vi "Prepare Control.vi"(7 "VolatusAPI":refnum<class "VolatusAPI.lvclass">, 8 "error in (no error)":errorcluster, 11 "ValveControl in":refnum<class "DigitalControl.lvclass">) -> (0 "error out":errorcluster, 3 "ValveControl out":refnum<class "DigitalControl.lvclass">)   [LabVIEW 2020, in "VolatusControl.lvlib" / "DigitalControl.lvclass"]
uses:
  DigitalControl.lvclass
  Volatus/VolatusAPI/VolatusAPI.lvclass
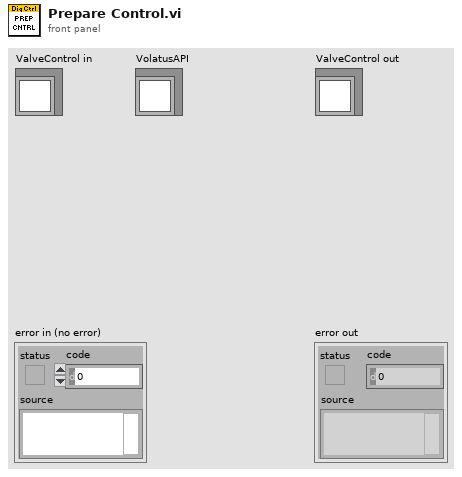
[diagram p1: front panel]
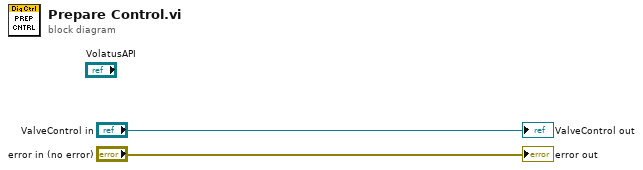
[diagram p0: block diagram]
diagram:
  "error out" <- "error in (no error)"
  "ValveControl out" <- "ValveControl in"
